vi "Blank2.vi"() -> ()   [LabVIEW 2020]
uses:
  <vilib>/DAQmx/read.llb/DAQmx Read.vi
  <vilib>/DAQmx/read.llb/DAQmx Read (Analog 1D DBL NChan 1Samp).vi
  <vilib>/DAQmx/miscellaneous.llb/DAQmx Fill In Error Info.vi
panel:
  in  "stop":bool
  out "data":dbl[](array[numeric]) format="%#_6p"
  in  "DAQmx Task Name":refnum<k21>
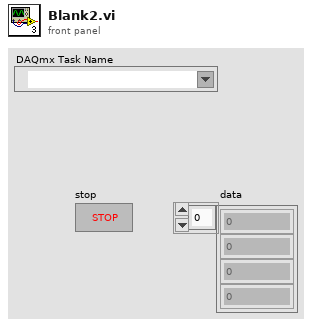
[diagram p1: front panel]
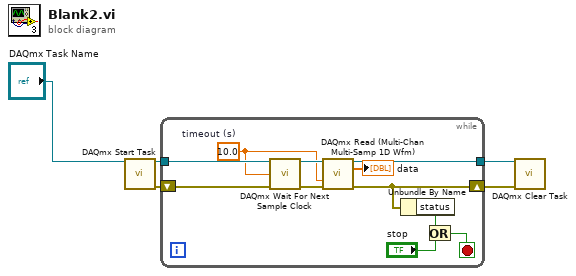
[diagram p0: block diagram]
diagram:
  n1 = call <vilib>:"DAQmx Start Task.vi"("task/channels in"="DAQmx Task Name") -> ("task out"=w5:refnum<k21>, "error out"=w4:errorcluster)  [unwired: 13 in]
  n2 = while {
    tunnel: w5 -> [w10]
    tunnel: [w11] -> w2
    shift-right: [w12] -> w3
    shift-left: w4 -> [w7]
    stop <- w13 stop-if-true
    w6 = 10.0  # timeout (s)
    n3 = call <vilib>:"DAQmx Wait For Next Sample Clock.vi"("task/channels in"=w10, "timeout (sec)"=w6, "error in"=w7) -> ("task out"=w9:refnum<k21>, "error out"=w8:errorcluster)  [unwired: 10 in, 1 out]
    n4 = call-poly "DAQmx Read (Multi-Chan Multi-Samp 1D Wfm).vi"("task/channels in"=w9, "timeout"=w6, "error in"=w8) -> ("task out"=w11:refnum<k21>, "data"=→"data":dbl[], "error out"=w12:errorcluster)  [unwired: 10 in]
    n5 = Unbundle By Name(w12) -> ("status"=w14:bool)
    n6 = Or(x=w14, y="stop") -> (x .or. y?=w13:bool)
  }
  n7 = call <vilib>:"DAQmx Clear Task.vi"("task in"=w2, "error in"=w3) -> ()  [unwired: 13 in, 1 out]
